vi "Host.vi"() -> ()   [LabVIEW 2022 SP3]
uses:
  <vilib>/FPGAPlugInAG/PXIe-7972R/niLvFpga_Open_PXIe-7972R.vi
  <vilib>/rvi/interface/common/dynamic/niFpgaDynamicAddResources.vi
  <vilib>/Utility/file.llb/Read Delimited Spreadsheet (DBL).vi
  <vilib>/Utility/error.llb/Error Cluster From Error Code.vi
  <vilib>/rvi/errors/niLvFpgaAdjustHostInterfaceError.vi
  <vilib>/FPGAPlugInAG/Dynamic/niLvFpga_Close_Dynamic.vi
  <vilib>/rvi/interface/nirviOpenFPGA/nirviOpenFPGA.xnode
  FPGA Bitfiles/untitledproject1_FPGATarget_7972RFPGAVIfirst_pcVphoSxrgk.lvbitx
  Phase_estimation.vi
  <vilib>/rvi/interface/nirviMethod/nirviMethod.xnode
  <vilib>/rvi/interface/nirviReadWriteControl/nirviReadWriteControl.xnode
  <vilib>/rvi/interface/nirviCloseFPGA/nirviCloseFPGA.xnode
  <vilib>/FPGAPlugInAG/Dynamic/niLvFpga_ReadFifo_Dynamic.vi
  <vilib>/rvi/errors/niLvFpgaMergeErrorWithErrorCode.vi
  <vilib>/FPGAPlugInAG/Dynamic/niLvFpga_WriteFifo_Dynamic.vi
  NiFpgaLv.dll
  <vilib>/rvi/interface/Simulation/niFpgaSimulationCallBeginRW.vi
panel:
  out "s? t:f":fxp<+/-,48,5>
  in  "White Noise Amplitude":u16
  in  "Add White Noise?":bool
  out "White Noise":waveform(dbl)(graph)
  out "error out 6":errorcluster
  out "Sgi":waveform(dbl)(graph)
  out "Sgphi":waveform(dbl)(graph)
  out "Phi":waveform(dbl)(graph)
  out "error out 4":errorcluster
  out "Sgi":waveform(dbl)(graph)
  out "error out 3":errorcluster
  in  "Memory\nDebug Mode":bool
  out "Data 2":fxp<+/-,18,-4>
  out "Data":fxp<+/-,18,-4>
  in  "Address":u32
  out "error out 2":errorcluster
  out "error out":errorcluster
  in  "Input? AI : Direct":bool
  out "Sgi":fxp<+/-,48,5>
  out "Sgphi":fxp<+/-,48,5>
  out "Phi":fxp<+/-,48,5>
  in  "Number of Elements":u32
  out "Weights Loaded":bool
  in  "psi_true":fxp<+/-,22,2>
  in  "DMA FIFO Output Resolution":u32
  out "Sgphi":waveform(dbl)(graph)
  in  "stop":bool
  out "Phi":waveform(dbl)(graph)
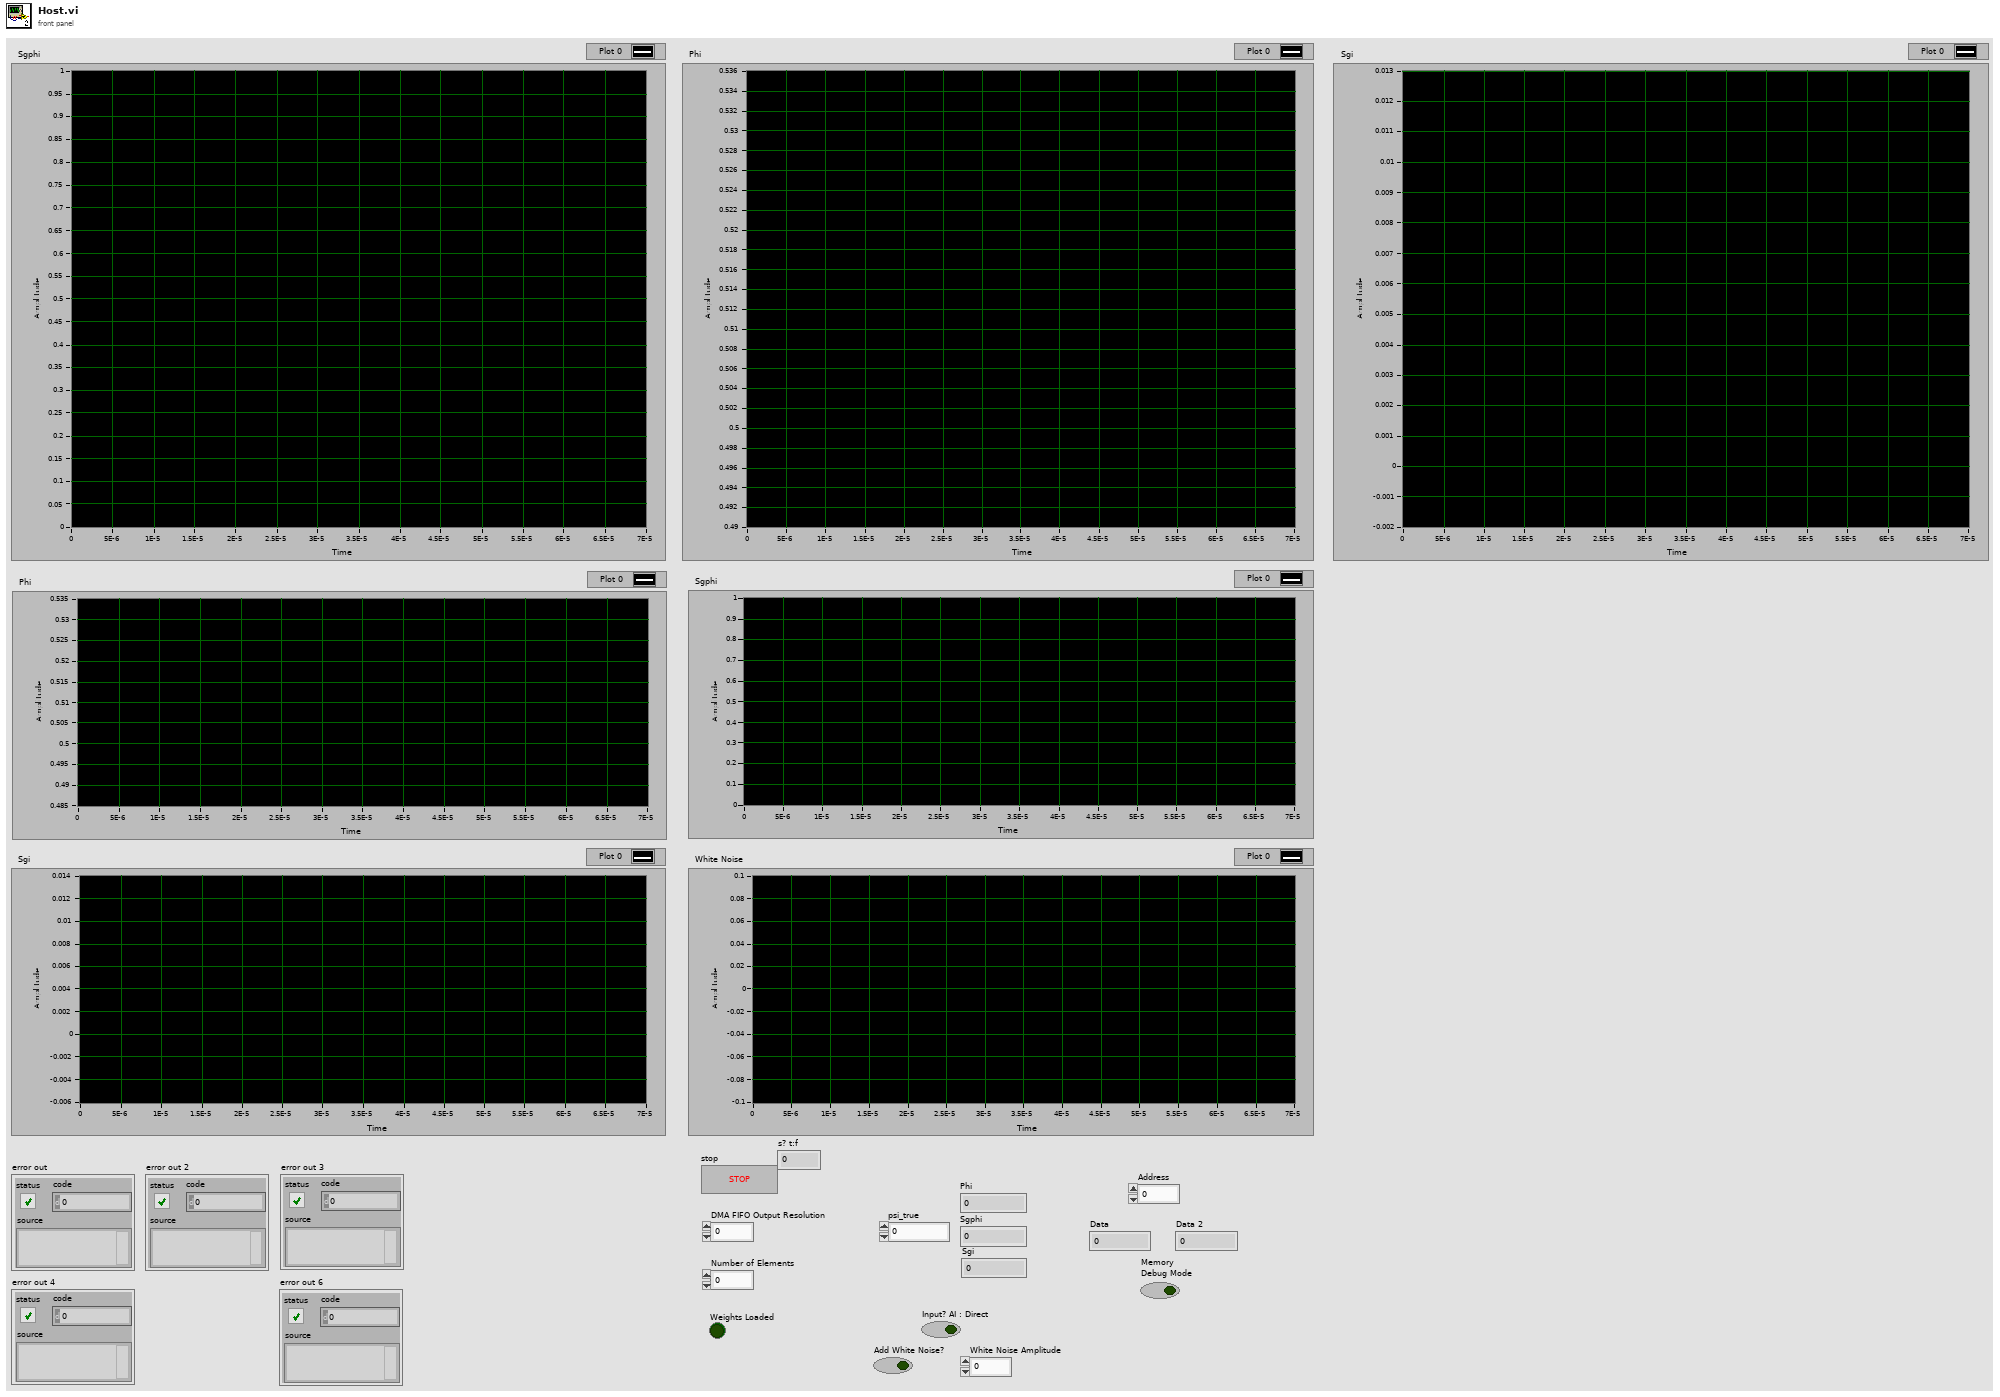
[diagram p1: front panel]
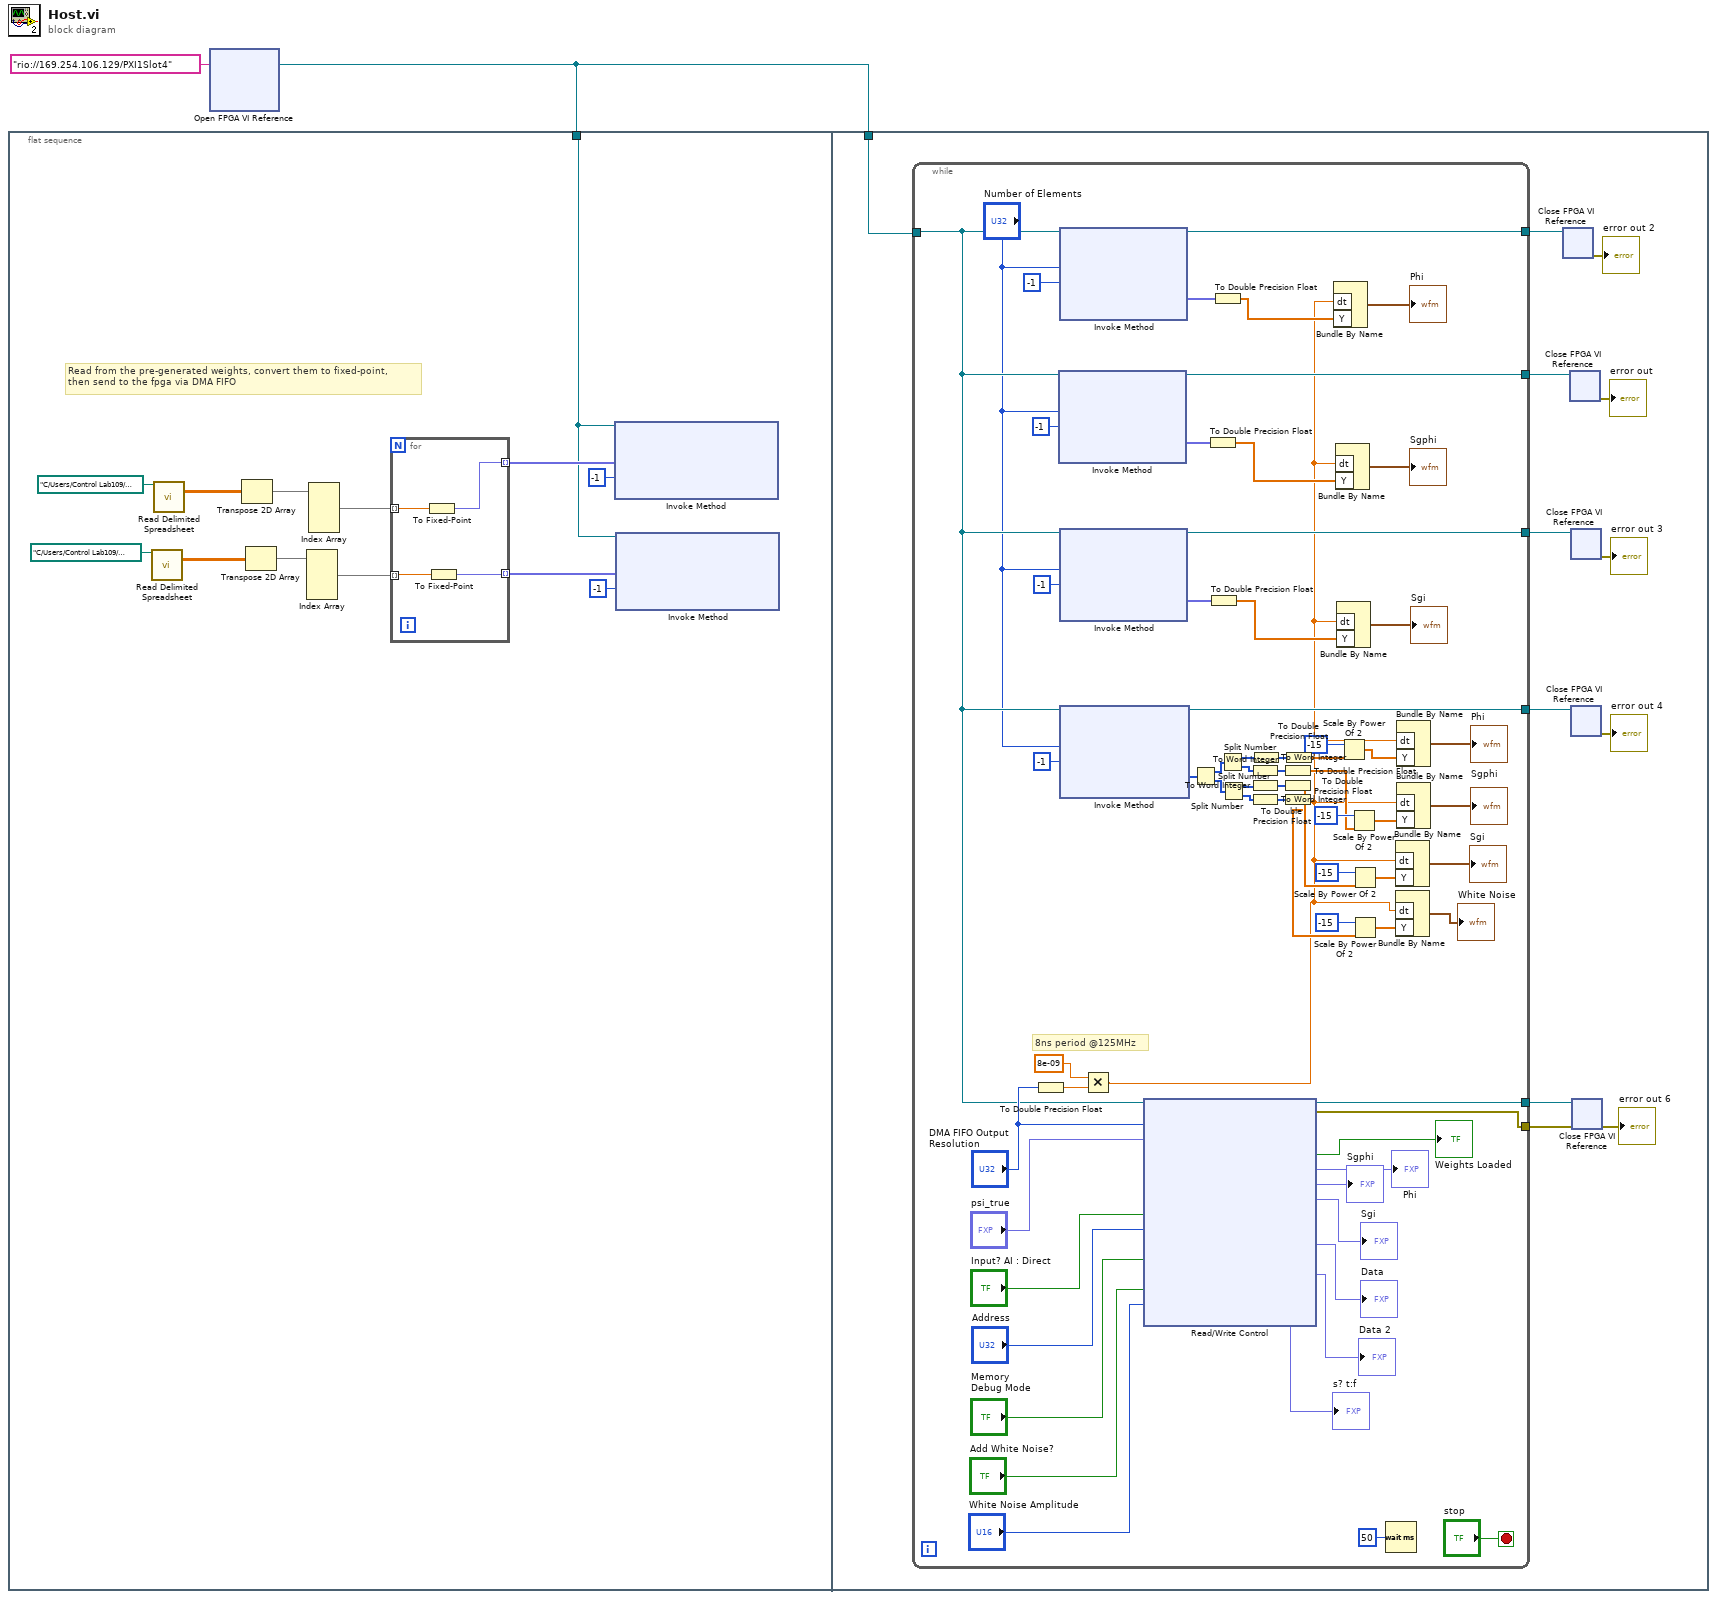
[diagram p0: block diagram]
diagram:
  n1 = flat-sequence {
    tunnel: w1 -> [w3]
    tunnel: w1 -> [w28]
    frame #0 {
      # "Read from the pre-generated weights, convert them to fixed-point,\nthen send to the fpga via DMA FIFO"
      n2 = call-poly <vilib>:"Read Delimited Spreadsheet.vi"("file path (dialog if empty)"=path "C:/Users/Control Lab109/Desktop/actual phase est/mark2_gdt.csv") -> ("all rows"=w14:dbl[][])  [unwired: 9 in, 5 out]
      n3 = call-poly <vilib>:"Read Delimited Spreadsheet.vi"("file path (dialog if empty)"=path "C:/Users/Control Lab109/Desktop/actual phase est/mark2_h.csv") -> ("all rows"=w15:dbl[][])  [unwired: 9 in, 5 out]
      n4 = Transpose 2D Array(2D array=w15) -> (transposed array=w11:dbl[][])
      n5 = Transpose 2D Array(2D array=w14) -> (transposed array=w7:dbl[][])
      n6 = Index Array(array=w7) -> (element #1=w6:dbl[])  [unwired: 4 in, 1 out]
      n7 = Index Array(array=w11) -> (element #1=w10:dbl[])  [unwired: 4 in, 1 out]
      n8 = for {
        tunnel: w10 -> [w19] mode=indexing
        tunnel: [w18] -> w4 mode=indexing
        tunnel: [w17] -> w5 mode=indexing
        tunnel: w6 -> [w16] mode=indexing
        n9 = To Fixed-Point(number=w19) -> (fixed-point=w18:fxp<+/-,18,-4>)  [unwired: 1 in]
        n10 = To Fixed-Point(number=w16) -> (fixed-point=w17:fxp<+/-,18,-4>)  [unwired: 1 in]
      }
      n11 = xnode "Invoke Method"("FPGA VI Reference In"=w3, "Data"=w4, "Timeout (ms)"=-1) -> ()  [unwired: 1 in, 3 out]
      n12 = xnode "Invoke Method"("FPGA VI Reference In"=w3, "Data"=w5, "Timeout (ms)"=-1) -> ()  [unwired: 1 in, 3 out]
    }
    frame #1 {
      n13 = while {
        tunnel: [w98] -> w31
        tunnel: [w91] -> w30
        tunnel: [w88] -> w29
        tunnel: w28 -> [w44]
        tunnel: [w72] -> w24
        tunnel: [w66] -> w23
        tunnel: [w40] -> w20
        stop <- "stop" stop-if-true
        # "8ns period @125MHz"
        n14 = To Double Precision Float(number="DMA FIFO Output Resolution") -> (double precision float=w69:dbl)
        n15 = xnode "Invoke Method"("FPGA VI Reference In"=w44, "Number of Elements"="Number of Elements", "Timeout (ms)"=-1) -> ("FPGA VI Reference Out"=w91:refnum<k20>, "Data"=w90:fxp<+/-,48,5>[])  [unwired: 1 in, 2 out]
        n16 = xnode "Invoke Method"("FPGA VI Reference In"=w44, "Number of Elements"="Number of Elements", "Timeout (ms)"=-1) -> ("FPGA VI Reference Out"=w98:refnum<k20>, "Data"=w96:fxp<+/-,48,5>[])  [unwired: 1 in, 2 out]
        n17 = xnode "Invoke Method"("FPGA VI Reference In"=w44, "Number of Elements"="Number of Elements", "Timeout (ms)"=-1) -> ("FPGA VI Reference Out"=w72:refnum<k20>, "Data"=w73:fxp<+/-,48,5>[])  [unwired: 1 in, 2 out]
        n18 = xnode "Invoke Method"("FPGA VI Reference In"=w44, "Number of Elements"="Number of Elements", "Timeout (ms)"=-1) -> ("FPGA VI Reference Out"=w66:refnum<k20>, "Data"=w64:u64[])  [unwired: 1 in, 2 out]
        n19 = Multiply(x=8e-09 ("dt"), y=w69) -> (x*y=w32:dbl)
        n20 = xnode "Read/Write Control"("FPGA VI Reference In"=w44, "DMA FIFO Output Resolution"="DMA FIFO Output Resolution", "psi_true"="psi_true", "Input? AI : Direct"="Input? AI : Direct", "Address"="Address", "Memory Debug Mode"="Memory\nDebug Mode", "Add White Noise?"="Add White Noise?", "White Noise Amplitude"="White Noise Amplitude") -> ("FPGA VI Reference Out"=w88:refnum<k20>, "error out"=w40:errorcluster, "Weights Loaded"=→"Weights Loaded":bool, "Phi"=→"Phi":fxp<+/-,48,5>, "Sgphi"=→"Sgphi":fxp<+/-,48,5>, "Sgi"=→"Sgi":fxp<+/-,48,5>, "Data"=→"Data":fxp<+/-,18,-4>, "Data 2"=→"Data 2":fxp<+/-,18,-4>, "s? t:f"=→"s? t:f":fxp<+/-,48,5>)  [unwired: 1 in]
        n21 = Split Number(x=w64) -> (hi(x)=w63:u32[], lo(x)=w62:u32[])
        n22 = To Double Precision Float(number=w90) -> (double precision float=w82:dbl[])
        n23 = To Double Precision Float(number=w73) -> (double precision float=w75:dbl[])
        n24 = To Double Precision Float(number=w96) -> (double precision float=w81:dbl[])
        n25 = Split Number(x=w63) -> (hi(x)=w59:u16[], lo(x)=w55:u16[])
        n26 = Split Number(x=w62) -> (hi(x)=w54:u16[], lo(x)=w36:u16[])
        n27 = To Word Integer(number=w55) -> (16bit integer=w57:i16[])
        n28 = To Word Integer(number=w54) -> (16bit integer=w56:i16[])
        n29 = To Word Integer(number=w36) -> (16bit integer=w35:i16[])
        n30 = To Word Integer(number=w59) -> (16bit integer=w58:i16[])
        n31 = To Double Precision Float(number=w57) -> (double precision float=w47:dbl[])
        n32 = To Double Precision Float(number=w56) -> (double precision float=w46:dbl[])
        n33 = To Double Precision Float(number=w35) -> (double precision float=w34:dbl[])
        n34 = To Double Precision Float(number=w58) -> (double precision float=w53:dbl[])
        n35 = Bundle By Name("dt"=w32, "Y"=w81) -> (→"Phi":waveform(dbl))  [unwired: 1 in]
        n36 = Bundle By Name("dt"=w32, "Y"=w82) -> (→"Sgphi":waveform(dbl))  [unwired: 1 in]
        n37 = Bundle By Name("dt"=w32, "Y"=w75) -> (→"Sgi":waveform(dbl))  [unwired: 1 in]
        n38 = Scale By Power Of 2(n=i16 -15, x=w53) -> (x*2^n=w48:dbl[])
        n39 = Scale By Power Of 2(n=i16 -15, x=w47) -> (x*2^n=w49:dbl[])
        n40 = Scale By Power Of 2(n=i16 -15, x=w46) -> (x*2^n=w45:dbl[])
        n41 = Scale By Power Of 2(n=i16 -15, x=w34) -> (x*2^n=w39:dbl[])
        n42 = Wait (ms)(milliseconds to wait=u32 50) -> ()  [unwired: 1 out]
        n43 = Bundle By Name("dt"=w32, "Y"=w45) -> (→"Sgi":waveform(dbl))  [unwired: 1 in]
        n44 = Bundle By Name("dt"=w32, "Y"=w39) -> (→"White Noise":waveform(dbl))  [unwired: 1 in]
        n45 = Bundle By Name("dt"=w32, "Y"=w48) -> (→"Phi":waveform(dbl))  [unwired: 1 in]
        n46 = Bundle By Name("dt"=w32, "Y"=w49) -> (→"Sgphi":waveform(dbl))  [unwired: 1 in]
      }
      n47 = xnode "Close FPGA VI Reference"("FPGA VI Reference In"=w31) -> ("error out"=→"error out 2":errorcluster)  [unwired: 1 in]
      n48 = xnode "Close FPGA VI Reference"("FPGA VI Reference In"=w30) -> ("error out"=→"error out":errorcluster)  [unwired: 1 in]
      n49 = xnode "Close FPGA VI Reference"("FPGA VI Reference In"=w24) -> ("error out"=→"error out 3":errorcluster)  [unwired: 1 in]
      n50 = xnode "Close FPGA VI Reference"("FPGA VI Reference In"=w23) -> ("error out"=→"error out 4":errorcluster)  [unwired: 1 in]
      n51 = xnode "Close FPGA VI Reference"("FPGA VI Reference In"=w29, "error in"=w20) -> ("error out"=→"error out 6":errorcluster)
    }
  }
  n52 = xnode "Open FPGA VI Reference"("resource name"=tag "rio://169.254.106.129/PXI1Slot4") -> ("FPGA VI Reference Out"=w1:refnum<k20>)  [unwired: 1 in, 1 out]
